vi "GetComparisonType.vi"(8 "error in":errorcluster, 11 "RangeMeasureLimit in":refnum<class "RangeMeasureLimit.lvclass">) -> (0 "error out":errorcluster, 2 "ComparisonType":T1, 3 "RangeMeasureLimit out":refnum<class "RangeMeasureLimit.lvclass">)   [LabVIEW 2021, in "ProligentXMLGenerator.lvlib" / "RangeMeasureLimit.lvclass"]
doc: "Real Measure Limit Comparison Type"
uses:
  RangeMeasureLimit.lvclass
  RangeMeasureLimit.lvclass/RangeMeasureLimit.ctl
  ComparisonType.ctl
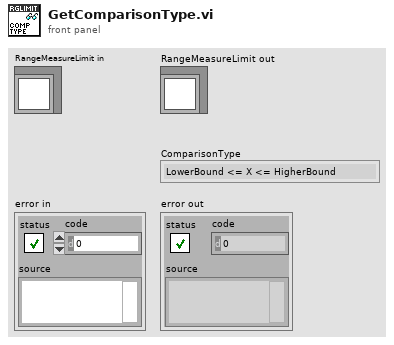
[diagram p1: front panel]
types:
  T1 = typedef "ProligentXMLGenerator.lvlib/RangeMeasureLimit.lvclass/ComparisonType.ctl" = enum16{"LowerBound <= X <= HigherBound", "LowerBound < X <= HigherBound", "LowerBound <= X < HigherBound", "LowerBound < X < HigherBound", "LowerBound <= X", "LowerBound < X", "X <= HigherBound", "X < HigherBound", "X == HigherBound", "X != HigherBound", "X <= LowerBound OR HigherBound <= X", "X < LowerBound OR HigherBound <= X", "X <= LowerBound OR HigherBound < X", "X < LowerBound OR HigherBound < X"}
  T2 = typedef "ProligentResultProcessor.lvlib/RangeMeasureLimit.lvclass/Data.ctl" = cluster{"ComparisonType":T3}
  T3 = typedef "ProligentResultProcessor.lvlib/RangeMeasureLimit.lvclass/ComparisonType.ctl" = enum16{"LowerBound <= X <= HigherBound", "LowerBound < X <= HigherBound", "LowerBound <= X < HigherBound", "LowerBound < X < HigherBound", "LowerBound <= X", "LowerBound < X", "X <= HigherBound", "X < HigherBound", "X == HigherBound", "X != HigherBound", "X <= LowerBound OR HigherBound <= X", "X < LowerBound OR HigherBound <= X", "X <= LowerBound OR HigherBound < X", "X < LowerBound OR HigherBound < X"}
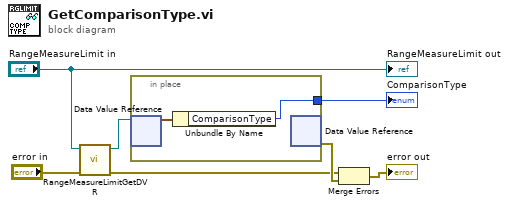
[diagram p0: block diagram]
diagram:
  n1 = call "RangeMeasureLimitGetDVR.vi"("error in"="error in", "RangeMeasureLimit"="RangeMeasureLimit in") -> ("error out"=w1:errorcluster, "DVRReference"=w6:refnum<data-value>)  [unwired: 8 in]
  n2 = in-place "In Place Element Structure" {
    in-place-border: [w8] -> w5
    n3 = in-place-dvr #1(w6) -> (w9:T2)  [unwired: 1 out]
    n4 = Unbundle By Name(w9) -> ("ComparisonType"=w8:T3)
    n5 = in-place-dvr #1() -> (w7:errorcluster)  [unwired: 1 in, 1 out]
  }
  "ComparisonType" <- w5
  n6 = Merge Errors(w1, w7) -> (→"error out":errorcluster)
  "RangeMeasureLimit out" <- "RangeMeasureLimit in"
